vi "File_cRIO Module.vi"(5 "Estado":bool=TRUE, 7 "Command":T2, 8 "error in (no error)":errorcluster, 9 "All Data":T1 {"CampoZ(T)" format="%.3e"; "CampoY(T)" format="%.3e"; "A.Input3(V)" format="%.3e"; "A.Input4(V)" format="%.3e"; "A.Input1(V)" format="%.3e"; "A.Input2(V)" format="%.3e"; "Temperatura(K)" format="%.3e"; "CampoX(T)" format="%.3e"; "Tiempo(min)" format="%.3e"}) -> (0 "error out":errorcluster, 2 "selected path":path)   [LabVIEW 2017]
uses:
  File_Module Control.ctl
  MEDIDA_cRIO_ZNB_AMI_DATOS.ctl
panel:
  out "Array":string[](array[string])
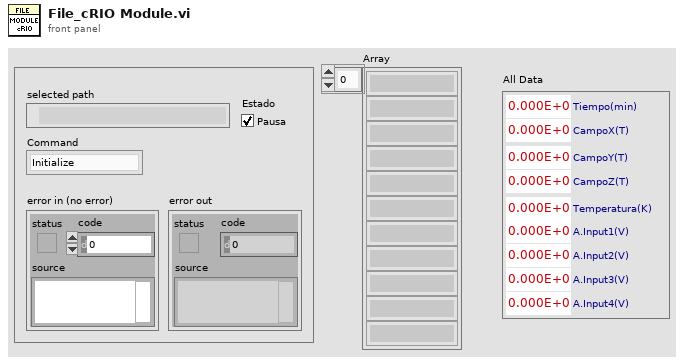
[diagram p1: front panel]
types:
  T1 = typedef "MEDIDA_cRIO_ZNB_AMI_DATOS.ctl" = cluster{"Tiempo(min)":dbl, "CampoX(T)":dbl, "CampoY(T)":dbl, "CampoZ(T)":dbl, "Temperatura(K)":dbl, "A.Input1(V)":dbl, "A.Input2(V)":dbl, "A.Input3(V)":dbl, "A.Input4(V)":dbl}
  T2 = typedef "File_Module Control.ctl" = enum16{"Initialize", "Save Head", "Save Data", "Shutdown"}
  T3 = enum16{"open", "replace", "create", "open or create", "replace or create", "replace or create with confirmation"}
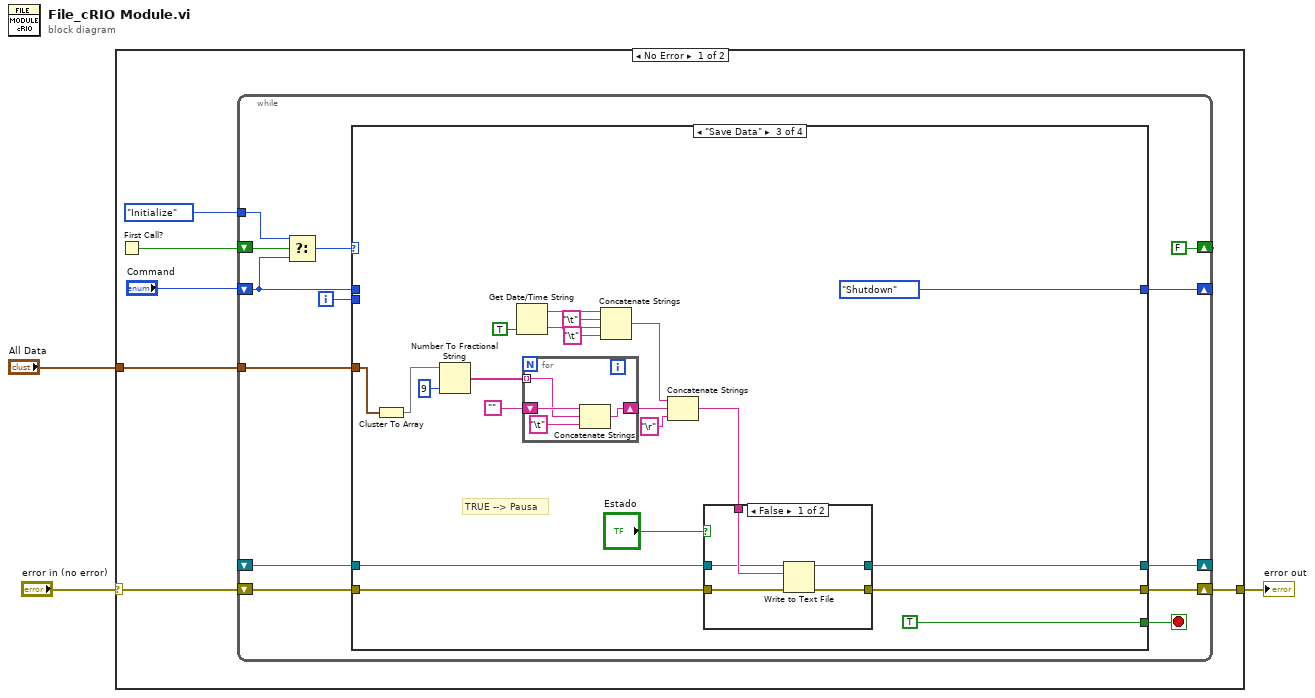
[diagram p0: block diagram]
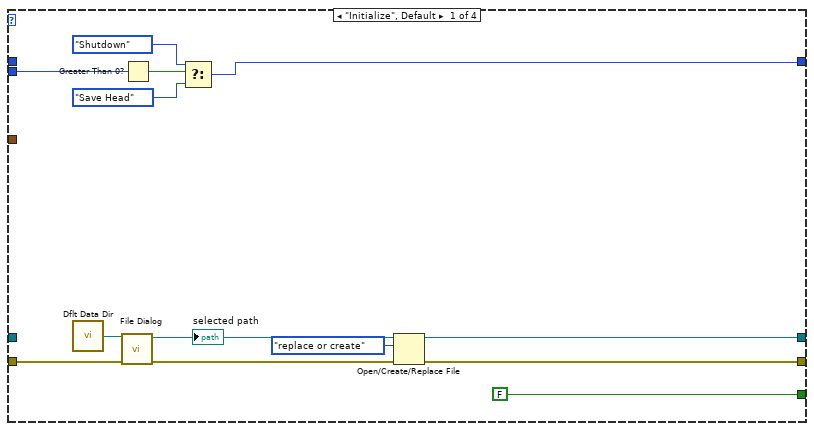
[diagram p2: hidden frame]
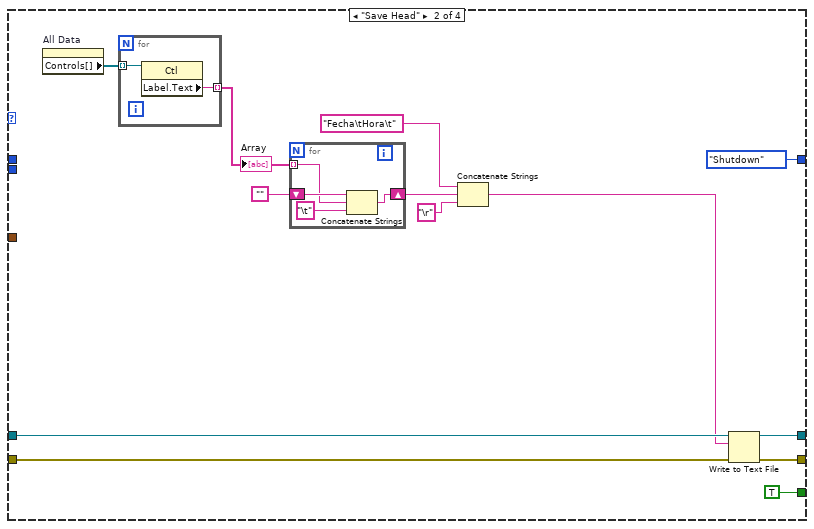
[diagram p3: hidden frame]
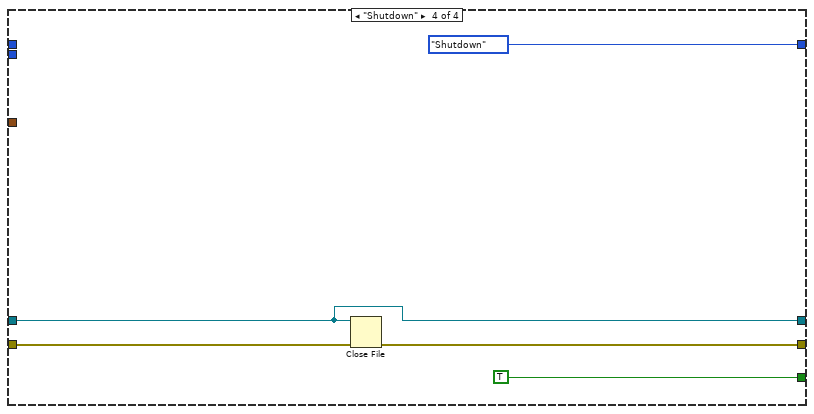
[diagram p5: hidden frame]
diagram:
  n1 = case shown="No Error" "error in (no error)" {
    selector: "error in (no error)" -> [w7 w92]
    tunnel: [w6 w92] -> w2
    tunnel: "All Data" -> [w4 _]
    frame No Error {
      n2 = First Call?() -> (First Call?: T/F=w9:bool)
      n3 = while {
        shift-right: [w14] -> _
        shift-left: "Command" -> [w15]
        shift-right: [w17] -> w6
        shift-left: w7 -> [w18]
        shift-right: [FALSE ("First Call?: T/F")] -> _
        shift-left: w9 -> [w22]
        tunnel: File_Module_Control."Initialize" ("t") -> [w21]
        shift-right: [w11] -> _
        shift-left: _ -> [w12]
        tunnel: w4 -> [w10]
        i -> [w13]
        stop <- w19 stop-if-true
        n4 = Select(t=w21, s=w22, f=w15) -> (s? t:f=w20:T2)
        n5 = case shown="\"Save Data\"" w20 {
          tunnel: [FALSE TRUE TRUE TRUE] -> w19
          tunnel: w18 -> [w28 w44 w70 w89]
          tunnel: [w24 w43 w69 w88] -> w17
          tunnel: w15 -> [_ _ _ _]
          tunnel: [w34 File_Module_Control."Shutdown" ("t") File_Module_Control."Shutdown" File_Module_Control."Shutdown"] -> w14
          tunnel: w13 -> [w32 _ _ _]
          tunnel: w12 -> [_ w46 w66 w87]
          tunnel: [w23 w45 w68 w87] -> w11
          tunnel: w10 -> [_ _ w56 _]
          frame "Initialize", Default {
            n6 = call <vilib>:"Dflt Data Dir.vi"() -> ("App:Default Data Directory"=w29:path)
            n7 = call "File Dialog"("start path"=w29, "error in"=w28) -> ("selected path"=w26:path, "error out"=w25:errorcluster)  [unwired: 10 in, 2 out]
            "selected path" <- w26
            n8 = Greater Than 0?(x=w32) -> (x > 0?=w31:bool)
            n9 = Select(t=File_Module_Control."Shutdown", s=w31, f=File_Module_Control."Save Head" ("t")) -> (s? t:f=w34:T2)
            n10 = Open/Create/Replace File(file path (use dialog)=w26, error in=w25, operation (0:open)=T3."replace or create") -> (refnum out=w23:refnum<file>, error out=w24:errorcluster)  [unwired: 3 in, 1 out]
          }
          frame "Save Head" {
            n11 = property on="All Data" class="Clust (strict)"() -> ("Controls[]"=w42:refnum<vi>[])  [unwired: 2 in, 2 out]
            n12 = for {
              tunnel: w42 -> [w54] mode=indexing
              tunnel: [w53] -> w37 mode=indexing
              n13 = property class="Ctl"(reference=w54) -> ("Label.Text"=w53:string)  [unwired: 1 in, 2 out]
            }
            "Array" <- w37
            n14 = for {
              tunnel: w37 -> [w51] mode=indexing
              shift-right: [w50] -> w41
              shift-left: "" -> [w52]
              n15 = Concatenate Strings(w52, w51, "\t" ("string")) -> (w50:string)
            }
            n16 = Concatenate Strings("Fecha\tHora\t" ("string"), w41, "\r" ("string")) -> (w36:string)
            n17 = Write to Text File(file (use dialog)=w46, text=w36, error in=w44) -> (refnum out=w45:refnum<file>, error out=w43:errorcluster)  [unwired: 1 in, 1 out]
          }
          frame "Save Data" {
            # "TRUE --> Pausa"
            n18 = Cluster To Array(cluster=w56) -> (array=w55:dbl[])
            n19 = Number To Fractional String(number=w55, precision (6)=i16 9) -> (F-format string=w59:string[])  [unwired: 2 in]
            n20 = Get Date/Time String(want seconds? (F)=TRUE) -> (date string=w62:string, time string=w61:string)  [unwired: 2 in]
            n21 = for {
              tunnel: w59 -> [w85] mode=indexing
              shift-right: [w84] -> w73
              shift-left: "" -> [w86]
              n22 = Concatenate Strings(w86, w85, "\t" ("string")) -> (w84:string)
            }
            n23 = Concatenate Strings(w62, "\t" ("string"), w61, "\t" ("string")) -> (w65:string)
            n24 = Concatenate Strings(w65, w73, "\r" ("string")) -> (w67:string)
            n25 = case shown="False" "Estado" {
              tunnel: w70 -> [w80 w81]
              tunnel: [w79 w81] -> w69
              tunnel: [w78 w82] -> w68
              tunnel: w67 -> [w77 _]
              tunnel: w66 -> [w76 w82]
              frame False {
                n26 = Write to Text File(file (use dialog)=w76, text=w77, error in=w80) -> (refnum out=w78:refnum<file>, error out=w79:errorcluster)  [unwired: 1 in, 1 out]
              }
              frame True {
              }
            }
          }
          frame "Shutdown" {
            n27 = Close File(refnum=w87, error in=w89) -> (error out=w88:errorcluster)  [unwired: 1 out]
          }
        }
      }
    }
    frame Error {
    }
  }
  "error out" <- w2
